vi "ErrorCluster to String.vi"(4 "error in (no error)":errorcluster) -> (0 "ErrorMSG":string, 1 "String":string)   [LabVIEW 2018]
doc: "Ver 1:00\nDESCRIPTION\nConverts Error cluster to string\n\nERROR HANDLING\nNone\n\n---------------------------------\nVERSION CONTROL\nVer 1:00 07/04/2000 ssdc"
uses:
  <vilib>/Utility/error.llb/DialogType.ctl
panel:
  # "Input"
  # "Output"
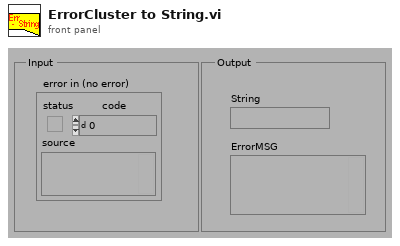
[diagram p1: front panel]
types:
  T1 = typedef "DialogType.ctl" = u16
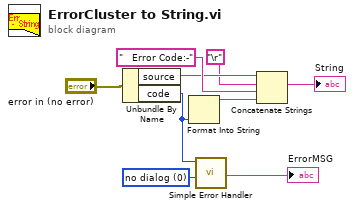
[diagram p0: block diagram]
diagram:
  w1 = T1 0 items=["no dialog", "OK message", "continue or stop message", "OK message + warnings", "continue/stop + warnings"] ("type of dialog (OK msg:1)")
  n1 = Unbundle By Name("error in (no error)") -> ("source"=w6:string, "code"=w2:i32)
  n2 = Format Into String(w2) -> (resulting string=w8:string)  [unwired: 3 in, 1 out]
  n3 = call <vilib>:"Simple Error Handler.vi"("error code (no error:0)"=w2, "type of dialog (OK msg:1)"=w1) -> ("message"=→"ErrorMSG":string)  [unwired: 3 in, 4 out]
  n4 = Concatenate Strings(w6, "\r", "   Error Code:-", w8) -> (→"String":string)
